vi "Mail Control V1.vi"() -> ()   [LabVIEW 2013]
uses:
  Global 1.vi
panel:
  out "MAIL SETTINGS IN":T1
  out "MAIL SELECT":T2
  in  "Stop Button":bool
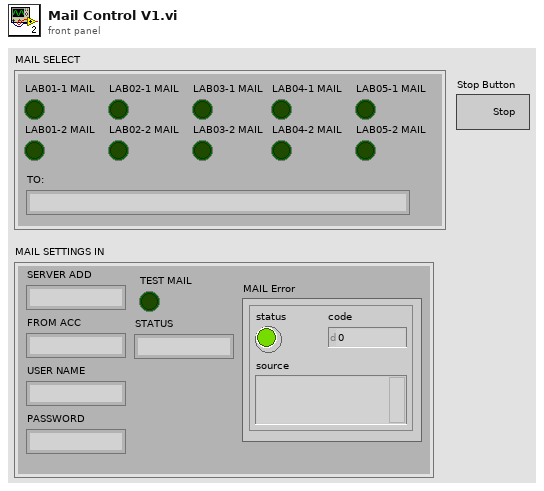
[diagram p1: front panel]
types:
  T1 = cluster{"SERVER ADD":string, "FROM ACC":string, "USER NAME":string, "PASSWORD":string, "TEST MAIL":bool, "STATUS":string, "MAIL Error":errorcluster}
  T2 = cluster{"LAB01-1 MAIL":bool, "LAB01-2 MAIL":bool, "LAB02-1 MAIL":bool, "LAB02-2 MAIL":bool, "LAB03-1 MAIL":bool, "LAB03-2 MAIL":bool, "LAB04-1 MAIL":bool, "LAB04-2 MAIL":bool, "LAB05-1 MAIL":bool, "LAB05-2 MAIL":bool, "TO:":string}
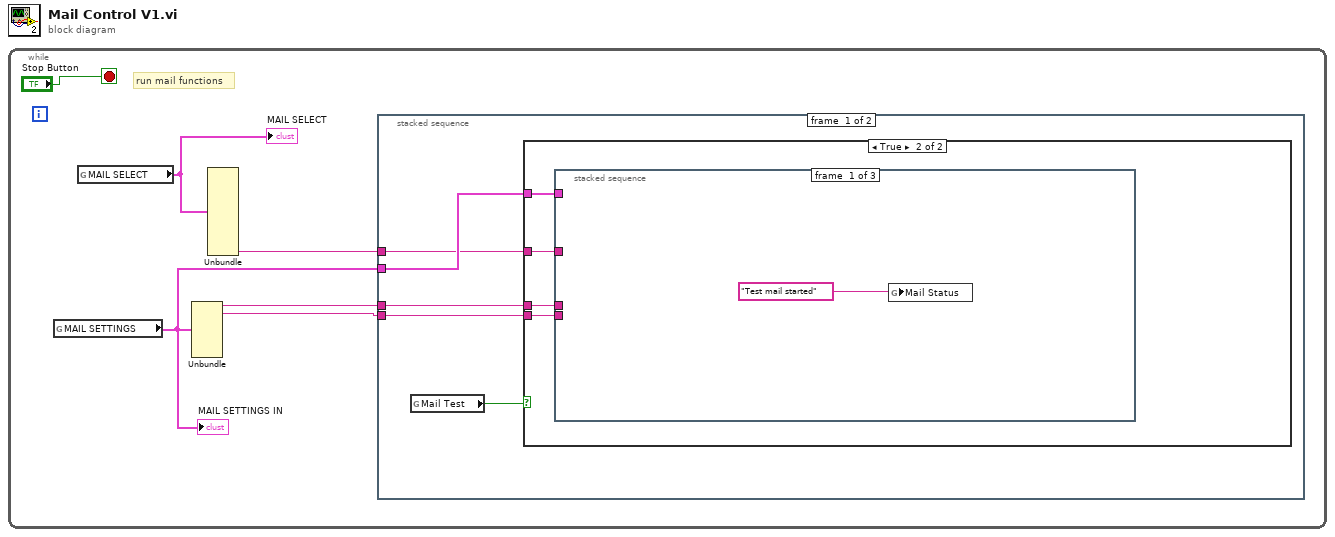
[diagram p0: block diagram]
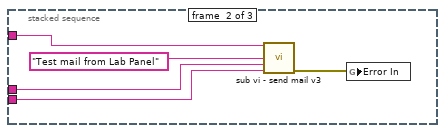
[diagram p3: hidden frame]
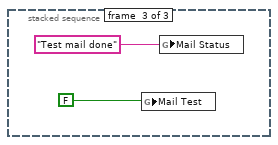
[diagram p4: hidden frame]
diagram:
  n1 = while {
    stop <- "Stop Button" stop-if-true
    # "run mail functions"
    n2 = global read "Global 1.vi" "MAIL SETTINGS"() -> (w4:T1)
    "MAIL SETTINGS IN" <- w4
    n3 = global read "Global 1.vi" "MAIL SELECT"() -> (w6:T2)
    "MAIL SELECT" <- w6
    n4 = Unbundle(w4) -> ("SERVER ADD"=w2:string, "FROM ACC"=w1:string)  [unwired: 5 out]
    n5 = Unbundle(w6) -> ("TO:"=w3:string)  [unwired: 10 out]
    n6 = stacked-sequence {
      tunnel: w4 -> [w11 _]
      tunnel: w3 -> [w10 _]
      tunnel: w2 -> [w9 _]
      tunnel: w1 -> [w8 _]
      frame #0 {
        n7 = global read "Global 1.vi" "Mail Test"() -> (w7:bool)
        n8 = case shown="True" w7 {
          tunnel: w11 -> [_ w12]
          tunnel: w10 -> [_ w15]
          tunnel: w9 -> [_ w14]
          tunnel: w8 -> [_ w13]
          frame False {
          }
          frame True {
            n9 = stacked-sequence {
              tunnel: w15 -> [_ w20 _]
              tunnel: w14 -> [_ w19 _]
              tunnel: w13 -> [_ w18 _]
              tunnel: w12 -> [_ _ _]
              frame #0 {
                n10 = global write "Global 1.vi" "Mail Status"("Test mail started") -> ()
              }
              frame #1 {
                n11 = call "sub vi - send mail v3.vi"("TO:"=w20, "subject"="Test mail from Lab Panel", "out going server"=w19, "from"=w18) -> ("error out"=w17:errorcluster)  [unwired: 11 in]
                n12 = global write "Global 1.vi" "Error In"(w17) -> ()
              }
              frame #2 {
                n13 = global write "Global 1.vi" "Mail Test"(FALSE) -> ()
                n14 = global write "Global 1.vi" "Mail Status"("Test mail done") -> ()
              }
            }
          }
        }
      }
      frame #1 {
      }
    }
  }
